vi "Teleop.vi"(10 "Match Info":T1={"Autonomous Elapsed Seconds"=0.0, "TeleOp Elapsed Seconds"=0.0, "Disabled Elapsed Seconds"=0.0, "Visited Autonomous"=FALSE, "Visited TeleOp"=FALSE, "Visited Disabled"=FALSE, "Autonomous Settings"={"Autonomous Style"=enum."Independent", "VI Refnum"=refnum}}, 11 "Call Context":T2) -> ()   [LabVIEW 2018]
doc: "This VI is called for each TeleOp packet received from the DS where the robot is not disabled. It is often used to read from the joysticks and update I/O or to update setpoints for timed control loops. It should complete and return within 20 milliseconds or it may miss DS packets."
uses:
  <vilib>/Rock Robotics/WPI/DriverStation/WPI_DriverStationDerivedRobotMode.ctl
  <vilib>/Rock Robotics/WPI/DriverStation/WPI_DriverStationMatch Info.ctl
  <vilib>/Rock Robotics/Network Tables/NT Read Boolean.vi
  <vilib>/Rock Robotics/Network Tables/NT Read Number.vi
  <vilib>/Rock Robotics/WPI/Utilities/WPI_GetSetVariantRefNum.vi
  <vilib>/Rock Robotics/Network Tables/NT Write Boolean.vi
  <vilib>/Rock Robotics/Network Tables/NT Write Boolean Array.vi
  <vilib>/Rock Robotics/Network Tables/NT Write Numeric Array.vi
  <vilib>/Rock Robotics/Network Tables/NT Read Numeric Array.vi
panel:
  in  "Motor Stall":dbl format="%#_13g"
  out "Sample Slider 0":dbl(slide) scale=0.0..5.0
  out "Sample Boolean 1":bool
  out "Sample Boolean 0":bool
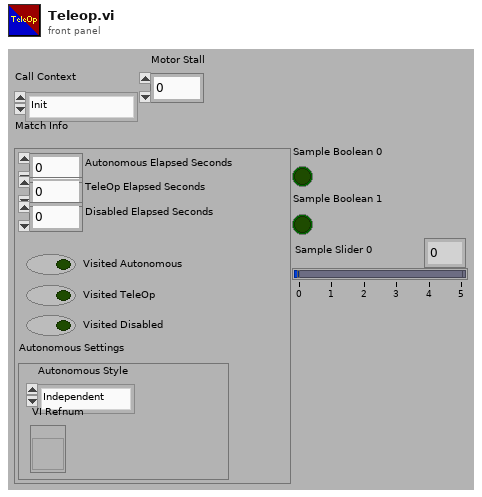
[diagram p1: front panel]
types:
  T1 = typedef "WPI_DriverStationMatch Info.ctl" = cluster{"Autonomous Elapsed Seconds":dbl, "TeleOp Elapsed Seconds":dbl, "Disabled Elapsed Seconds":dbl, "Visited Autonomous":bool, "Visited TeleOp":bool, "Visited Disabled":bool, "Autonomous Settings":cluster{"Autonomous Style":enum16{"Iterative", "Independent"}, "VI Refnum":refnum<vi>}}
  T2 = typedef "WPI_DriverStationDerivedRobotMode.ctl" = enum16{"Init", "Execute", "Stop"}
  T3 = typedef "WPI_JoystickDevRef.ctl" = cluster{"Device":T4}
  T4 = typedef "WPI_JoystickDeviceEnum.ctl" = enum16{"USB 0", "USB 1", "USB 2", "USB 3", "USB 4", "USB 5"}
  T5 = typedef "WPI_MotorControlDeviceRef.ctl" = cluster{"DeviceStatus":errorcluster, "Type":T6, "PWM":cluster{"PWM Channel":T7, "DeadBand":T8}, "CAN":cluster{"Device Number":u8, "SetOutput VI Ref":variant, "GetOutput VI Ref":variant, "Enable VI Ref":variant, "Disable VI Ref":variant, "Data":variant}, "Invert":bool, "DIO PWM":cluster{"PWM \"Enable\" Channel":T7, "DIOChannel":T9, "PWM Rate":dbl}}
  T6 = typedef "WPI_MotorControlType.ctl" = enum16{"PWM", "CAN", "DIO PWM"}
  T7 = typedef "FPGA_DIOPWMChannel.ctl" = enum8{"PWM 0", "PWM 1", "PWM 2", "PWM 3", "PWM 4", "PWM 5", "PWM 6", "PWM 7", "PWM 8", "PWM 9", "PWM MXP 0", "PWM MXP 1", "PWM MXP 2", "PWM MXP 3", "PWM MXP 4", "PWM MXP 5", "PWM MXP 6", "PWM MXP 7", "PWM MXP 8", "PWM MXP 9", "Invalid"}
  T8 = typedef "WPI_PWMDeadband.ctl" = cluster{"Name":string, "maxPositivePwm":i32, "minPositivePwm":i32, "centerPwm":i32, "maxNegativePwm":i32, "minNegativePwm":i32, "angularRange":u16}
  T9 = typedef "FPGA_DIOChannel.ctl" = enum8{"DIO 0", "DIO 1", "DIO 2", "DIO 3", "DIO 4", "DIO 5", "DIO 6", "DIO 7", "DIO 8", "DIO 9", "DIO MXP 0", "DIO MXP 1", "DIO MXP 2", "DIO MXP 3", "DIO MXP 4", "DIO MXP 5", "DIO MXP 6", "DIO MXP 7", "DIO MXP 8", "DIO MXP 9", "DIO MXP 10", "DIO MXP 11", "DIO MXP 12", "DIO MXP 13", "DIO MXP 14", "DIO MXP 15", "SPI Port CS1", "SPI Port CS2", "SPI Port CS3", "SPI Port MISO", "SPI Port MOSI", "Invalid"}
  T10 = typedef "WPI_RobotDriveDevRef.ctl" = cluster{"DevStatus":errorcluster, "Motors[]":T5[], "Square Inputs":bool, "Max Output":dbl}
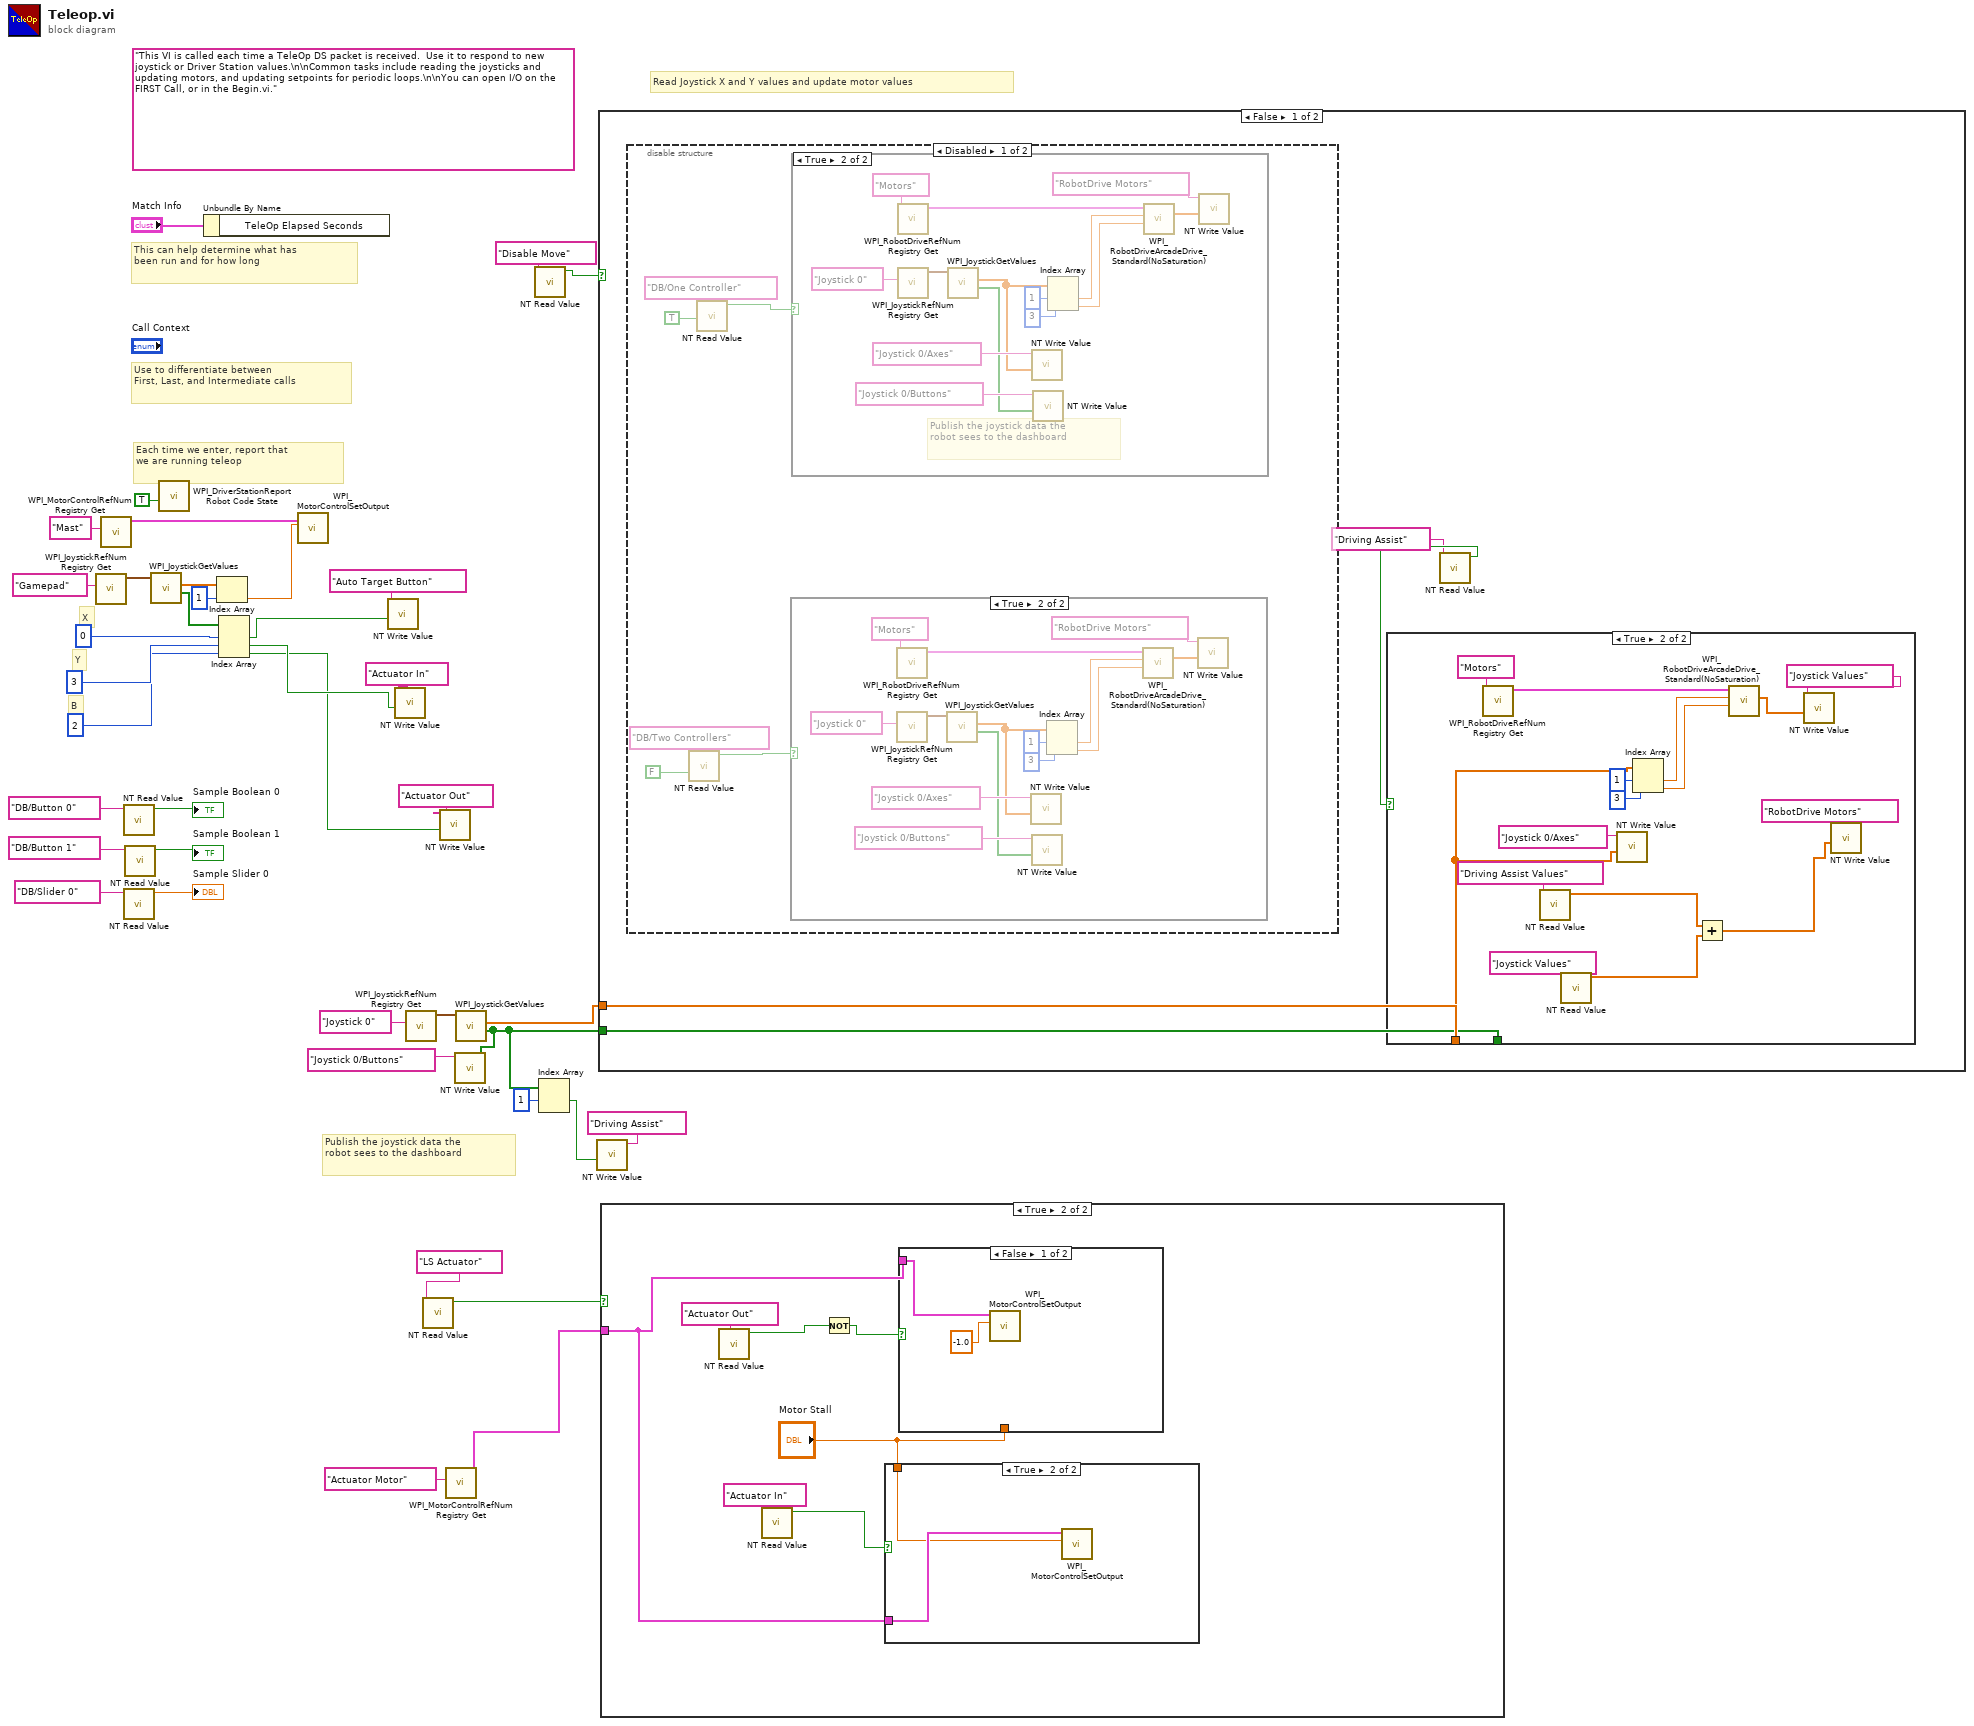
[diagram p0: block diagram]
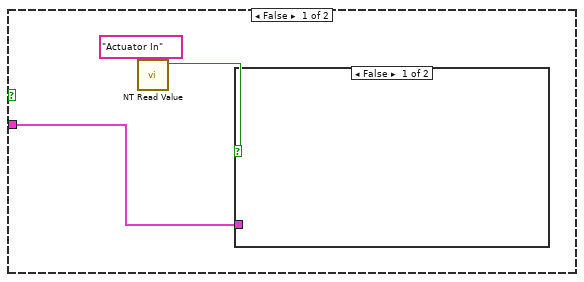
[diagram p2: hidden frame]
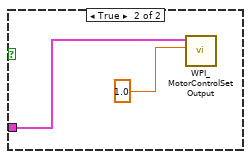
[diagram p3: hidden frame]
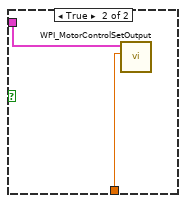
[diagram p5: hidden frame]
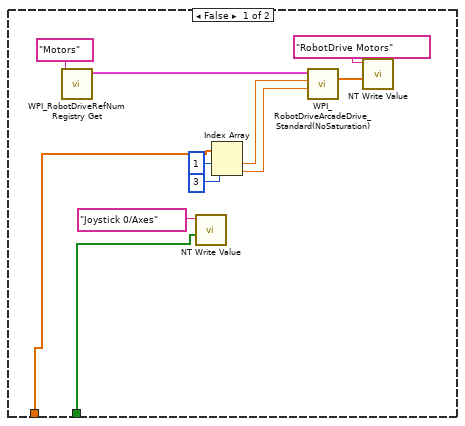
[diagram p6: hidden frame]
diagram:
  (unwired) "This VI is called each time a TeleOp DS packet is received.  Use it to respond to new joystick or Driver Station values.\n\nCommon tasks include reading the joysticks and updating motors, and updating setpoints for periodic loops.\n\nYou can open I/O on the FIRST Call, or in the Begin.vi."
  # "Publish the joystick data the\nrobot sees to the dashboard"
  # "B"
  # "X"
  # "Y"
  # "Each time we enter, report that\nwe are running teleop"
  # "Use to differentiate between\nFirst, Last, and Intermediate calls"
  # "This can help determine what has\nbeen run and for how long"
  # "Read Joystick X and Y values and update motor values"
  n1 = call <vilib>:"WPI_JoystickRefNum Registry Get.vi"("refnum name"="Gamepad") -> ("JoystickDevRef"=w28:T3)  [unwired: 9 in, 1 out]
  n2 = call <vilib>:"WPI_MotorControlRefNum Registry Get.vi"("refnum name"="Mast") -> ("MotorControlDevRef"=w30:T5)  [unwired: 9 in, 1 out]
  n3 = call-poly <vilib>:"NT Read Value.vi"("Name"="DB/Button 0" ("refnum name")) -> ("Boolean"=→"Sample Boolean 0":bool)  [unwired: 9 in, 1 out]
  n4 = call-poly <vilib>:"NT Read Value.vi"("Name"="DB/Slider 0" ("refnum name")) -> ("Numeric"=→"Sample Slider 0":dbl)  [unwired: 9 in, 1 out]
  n5 = call-poly <vilib>:"NT Read Value.vi"("Name"="DB/Button 1" ("refnum name")) -> ("Boolean"=→"Sample Boolean 1":bool)  [unwired: 9 in, 1 out]
  n6 = call <vilib>:"WPI_JoystickGetValues.vi"("JoystickDevRef"=w28) -> ("Buttons"=w22:bool[], "Axes"=w27:dbl[])  [unwired: 6 in, 3 out]
  n7 = call <vilib>:"WPI_DriverStationReport Robot Code State.vi"("TeleOp"=TRUE ("Autonomous")) -> ()  [unwired: 10 in, 1 out]
  n8 = Unbundle By Name("Match Info") -> ()  [unwired: 1 out]
  n9 = Index Array(array=w27, index=1) -> (element=w26:dbl)
  n10 = Index Array(array=w22, index #1=0 ("index"), index #2=3 ("index"), index #3=2 ("index")) -> (element #1=w20:bool, element #2=w14:bool, element #3=w11:bool)
  n11 = call <vilib>:"WPI_MotorControlSetOutput.vi"("Output"=w26, "MotorControlDevRef"=w30) -> ()  [unwired: 7 in, 3 out]
  n12 = call-poly <vilib>:"NT Write Value.vi"("Boolean"=w20, "Name"="Auto Target Button") -> ()  [unwired: 9 in, 1 out]
  n13 = call-poly <vilib>:"NT Write Value.vi"("Boolean"=w14, "Name"="Actuator In") -> ()  [unwired: 9 in, 1 out]
  n14 = call <vilib>:"WPI_JoystickRefNum Registry Get.vi"("refnum name"="Joystick 0") -> ("JoystickDevRef"=w8:T3)  [unwired: 1 in, 9 out]
  n15 = call-poly <vilib>:"NT Read Value.vi"("Name"="LS Actuator") -> ("Boolean"=w17:bool)  [unwired: 9 in, 1 out]
  n16 = call-poly <vilib>:"NT Write Value.vi"("Boolean"=w11, "Name"="Actuator Out") -> ()  [unwired: 9 in, 1 out]
  n17 = call <vilib>:"WPI_MotorControlRefNum Registry Get.vi"("refnum name"="Actuator Motor") -> ("MotorControlDevRef"=w9:T5)  [unwired: 9 in, 1 out]
  n18 = call <vilib>:"WPI_JoystickGetValues.vi"("JoystickDevRef"=w8) -> ("Buttons"=w4:bool[], "Axes"=w6:dbl[])  [unwired: 6 in, 3 out]
  n19 = call-poly <vilib>:"NT Write Value.vi"("Boolean Array"=w4, "Name"="Joystick 0/Buttons") -> ()  [unwired: 9 in, 1 out]
  n20 = call-poly <vilib>:"NT Read Value.vi"("Name"="Disable Move") -> ("Boolean"=w24:bool)  [unwired: 9 in, 1 out]
  n21 = Index Array(array=w4, index #1=1 ("index")) -> (element #1=w2:bool)  [unwired: 1 in, 1 out]
  n22 = call-poly <vilib>:"NT Write Value.vi"("Boolean"=w2, "Name"="Driving Assist") -> ()  [unwired: 9 in, 1 out]
  n23 = case shown="False" w24 {
    tunnel: w4 -> [w42 _]
    tunnel: w6 -> [w43 _]
    frame False {
      n24 = disable-structure shown="Disabled" {
        frame Disabled {
          n25 = call-poly <vilib>:"NT Read Value.vi"("Default Value"=FALSE, "Name"="DB/Two Controllers") -> ("Boolean"=w74:bool)  [unwired: 8 in, 1 out]
          n26 = call-poly <vilib>:"NT Read Value.vi"("Default Value"=TRUE, "Name"="DB/One Controller") -> ("Boolean"=w76:bool)  [unwired: 8 in, 1 out]
          n27 = case shown="True" w74 {
            frame False {
            }
            frame True {
              n28 = call <vilib>:"WPI_RobotDriveRefNum Registry Get.vi"("refnum name"="Motors") -> ("RobotDriveDevRef"=w89:T10)  [unwired: 1 in, 9 out]
              n29 = call <vilib>:"WPI_JoystickRefNum Registry Get.vi"("refnum name"="Joystick 0") -> ("JoystickDevRef"=w87:T3)  [unwired: 1 in, 9 out]
              n30 = call <vilib>:"WPI_JoystickGetValues.vi"("JoystickDevRef"=w87) -> ("Buttons"=w82:bool[], "Axes"=w83:dbl[])  [unwired: 6 in, 3 out]
              n31 = call-poly <vilib>:"NT Write Value.vi"("Numeric Array"=w83, "Name"="Joystick 0/Axes") -> ()  [unwired: 9 in, 1 out]
              n32 = call-poly <vilib>:"NT Write Value.vi"("Boolean Array"=w82, "Name"="Joystick 0/Buttons") -> ()  [unwired: 9 in, 1 out]
              n33 = Index Array(array=w83, index #1=1 ("index"), index #2=3 ("index")) -> (element #1=w88:dbl, element #2=w86:dbl)
              n34 = call <vilib>:"WPI_RobotDriveArcadeDrive_Standard(NoSaturation).vi"("Y axis value"=w86, "X axis value"=w88, "RobotDriveDevRef"=w89) -> ("Motor Values"=w81:dbl[])  [unwired: 1 in, 7 out]
              n35 = call-poly <vilib>:"NT Write Value.vi"("Numeric Array"=w81, "Name"="RobotDrive Motors") -> ()  [unwired: 9 in, 1 out]
            }
          }
          n36 = case shown="True" w76 {
            frame False {
            }
            frame True {
              # "Publish the joystick data the\nrobot sees to the dashboard"
              n37 = call <vilib>:"WPI_RobotDriveRefNum Registry Get.vi"("refnum name"="Motors") -> ("RobotDriveDevRef"=w103:T10)  [unwired: 1 in, 9 out]
              n38 = call <vilib>:"WPI_JoystickRefNum Registry Get.vi"("refnum name"="Joystick 0") -> ("JoystickDevRef"=w101:T3)  [unwired: 1 in, 9 out]
              n39 = call <vilib>:"WPI_JoystickGetValues.vi"("JoystickDevRef"=w101) -> ("Buttons"=w96:bool[], "Axes"=w97:dbl[])  [unwired: 6 in, 3 out]
              n40 = call-poly <vilib>:"NT Write Value.vi"("Numeric Array"=w97, "Name"="Joystick 0/Axes") -> ()  [unwired: 9 in, 1 out]
              n41 = call-poly <vilib>:"NT Write Value.vi"("Boolean Array"=w96, "Name"="Joystick 0/Buttons") -> ()  [unwired: 9 in, 1 out]
              n42 = Index Array(array=w97, index #1=1 ("index"), index #2=3 ("index")) -> (element #1=w102:dbl, element #2=w100:dbl)
              n43 = call <vilib>:"WPI_RobotDriveArcadeDrive_Standard(NoSaturation).vi"("Y axis value"=w100, "X axis value"=w102, "RobotDriveDevRef"=w103) -> ("Motor Values"=w95:dbl[])  [unwired: 1 in, 7 out]
              n44 = call-poly <vilib>:"NT Write Value.vi"("Numeric Array"=w95, "Name"="RobotDrive Motors") -> ()  [unwired: 9 in, 1 out]
            }
          }
        }
        frame Enabled {
        }
      }
      n45 = call-poly <vilib>:"NT Read Value.vi"("Name"="Driving Assist") -> ("Boolean"=w41:bool)  [unwired: 9 in, 1 out]
      n46 = case shown="True" w41 {
        tunnel: w43 -> [w45 w63]
        tunnel: w42 -> [w44 _]
        frame False {
          n47 = call <vilib>:"WPI_RobotDriveRefNum Registry Get.vi"("refnum name"="Motors") -> ("RobotDriveDevRef"=w53:T10)  [unwired: 1 in, 9 out]
          n48 = call-poly <vilib>:"NT Write Value.vi"("Boolean Array"=w44, "Name"="Joystick 0/Axes") -> ()  [unwired: 9 in, 1 out]
          n49 = Index Array(array=w45, index #1=1 ("index"), index #2=3 ("index")) -> (element #1=w52:dbl, element #2=w51:dbl)
          n50 = call <vilib>:"WPI_RobotDriveArcadeDrive_Standard(NoSaturation).vi"("Y axis value"=w51, "X axis value"=w52, "RobotDriveDevRef"=w53) -> ("Motor Values"=w49:dbl[])  [unwired: 1 in, 7 out]
          n51 = call-poly <vilib>:"NT Write Value.vi"("Numeric Array"=w49, "Name"="RobotDrive Motors") -> ()  [unwired: 9 in, 1 out]
        }
        frame True {
          n52 = call <vilib>:"WPI_RobotDriveRefNum Registry Get.vi"("refnum name"="Motors") -> ("RobotDriveDevRef"=w69:T10)  [unwired: 1 in, 9 out]
          n53 = call-poly <vilib>:"NT Read Value.vi"("Name"="Driving Assist Values") -> ("Numeric Array"=w58:dbl[])  [unwired: 9 in, 1 out]
          n54 = call-poly <vilib>:"NT Read Value.vi"("Name"="Joystick Values") -> ("Numeric Array"=w57:dbl[])  [unwired: 9 in, 1 out]
          n55 = call-poly <vilib>:"NT Write Value.vi"("Numeric Array"=w63, "Name"="Joystick 0/Axes") -> ()  [unwired: 9 in, 1 out]
          n56 = Index Array(array=w63, index #1=1 ("index"), index #2=3 ("index")) -> (element #1=w68:dbl, element #2=w67:dbl)
          n57 = Add(x=w58, y=w57) -> (x+y=w55:dbl[])
          n58 = call <vilib>:"WPI_RobotDriveArcadeDrive_Standard(NoSaturation).vi"("Y axis value"=w67, "X axis value"=w68, "RobotDriveDevRef"=w69) -> ("Motor Values"=w61:dbl[])  [unwired: 1 in, 7 out]
          n59 = call-poly <vilib>:"NT Write Value.vi"("Numeric Array"=w61, "Name"="Joystick Values") -> ()  [unwired: 9 in, 1 out]
          n60 = call-poly <vilib>:"NT Write Value.vi"("Numeric Array"=w55, "Name"="RobotDrive Motors") -> ()  [unwired: 9 in, 1 out]
        }
      }
    }
    frame True {
    }
  }
  n61 = case shown="True" w17 {
    tunnel: w9 -> [w105 w111]
    frame False {
      n62 = call-poly <vilib>:"NT Read Value.vi"("Name"="Actuator In") -> ("Boolean"=w106:bool)  [unwired: 9 in, 1 out]
      n63 = case shown="False" w106 {
        tunnel: w105 -> [_ w108]
        frame False {
        }
        frame True {
          n64 = call <vilib>:"WPI_MotorControlSetOutput.vi"("Output"=1.0, "MotorControlDevRef"=w108) -> ()  [unwired: 7 in, 3 out]
        }
      }
    }
    frame True {
      n65 = call-poly <vilib>:"NT Read Value.vi"("Name"="Actuator Out") -> ("Boolean"=w115:bool)  [unwired: 9 in, 1 out]
      n66 = call-poly <vilib>:"NT Read Value.vi"("Name"="Actuator In") -> ("Boolean"=w112:bool)  [unwired: 9 in, 1 out]
      n67 = Not(x=w115) -> (.not. x?=w114:bool)
      n68 = case shown="True" w112 {
        tunnel: w111 -> [_ w118]
        tunnel: "Motor Stall" -> [_ w117]
        frame False {
        }
        frame True {
          n69 = call <vilib>:"WPI_MotorControlSetOutput.vi"("Output"=w117, "MotorControlDevRef"=w118) -> ()  [unwired: 7 in, 3 out]
        }
      }
      n70 = case shown="False" w114 {
        tunnel: w111 -> [w120 w122]
        tunnel: "Motor Stall" -> [_ w121]
        frame False {
          n71 = call <vilib>:"WPI_MotorControlSetOutput.vi"("Output"=-1.0, "MotorControlDevRef"=w120) -> ()  [unwired: 7 in, 3 out]
        }
        frame True {
          n72 = call <vilib>:"WPI_MotorControlSetOutput.vi"("Output"=w121, "MotorControlDevRef"=w122) -> ()  [unwired: 7 in, 3 out]
        }
      }
    }
  }
